vi "Error_And_Status_Test.vi"() -> ()   [LabVIEW 2017]
uses:
  Classes/ADCP.lvclass
panel:
  out "Test conditions / results":T1(array[cluster])
  in  "ADCP Session Parameters":T2
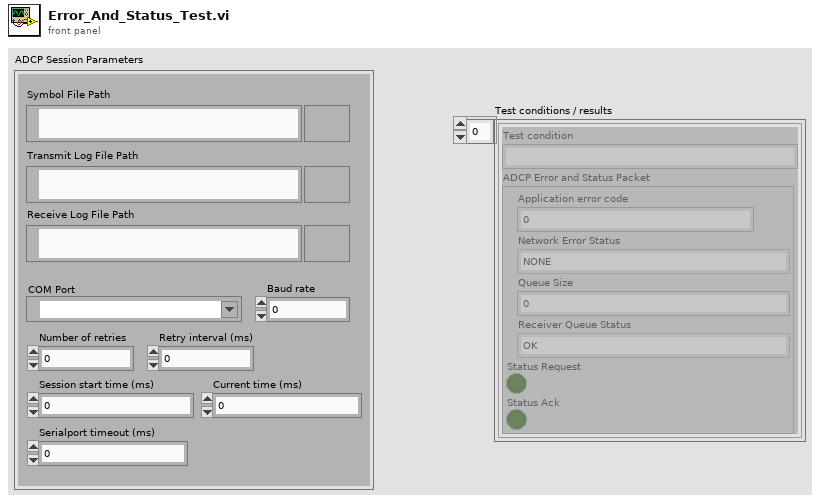
[diagram p1: front panel]
types:
  T1 = cluster{"Test condition":string, "ADCP Error and Status Packet":cluster{"Application error code":u16, "Network Error Status":enum16{"NONE", "CONNECTION_ALREADY_OPEN", "CONNECTION_ALREADY_CLOSED", "INVALID_FRAME_REQUEST"}, "Queue Size":u16, "Receiver Queue Status":enum16{"OK", "EMPTY", "FULL"}, "Status Request":bool, "Status Ack":bool}}[]
  T2 = cluster{"Symbol File Path":path, "Transmit Log File Path":path, "Receive Log File Path":path, "COM Port":refnum<visa-resource-name>, "Baud rate":u32, "Number of retries":u16, "Retry interval (ms)":u16, "Session start time (ms)":u32, "Current time (ms)":u32, "Serialport timeout (ms)":u32}
  T3 = cluster{"Application error code":u16, "Network Error Status":enum16{"NONE", "CONNECTION_ALREADY_OPEN", "CONNECTION_ALREADY_CLOSED", "INVALID_FRAME_REQUEST"}, "Queue Size":u16, "Receiver Queue Status":enum16{"OK", "EMPTY", "FULL"}, "Status Request":bool, "Status Ack":bool}
  T4 = cluster{"Application error code":u16, "Network Error Status":enum16{"NONE", "CONNECTION_ALREADY_OPEN", "CONNECTION_ALREADY_CLOSED", "INVALID_FRAME_REQUEST"}, "Queue Size":u16, "Receiver Queue Status":enum16{"OK", "EMPTY", "FULL"}, "Status Request":bool, "Status Ack":bool}[]
  T5 = cluster{"Test condition":string, "ADCP Error and Status Packet":cluster{"Application error code":u16, "Network Error Status":enum16{"NONE", "CONNECTION_ALREADY_OPEN", "CONNECTION_ALREADY_CLOSED", "INVALID_FRAME_REQUEST"}, "Queue Size":u16, "Receiver Queue Status":enum16{"OK", "EMPTY", "FULL"}, "Status Request":bool, "Status Ack":bool}}
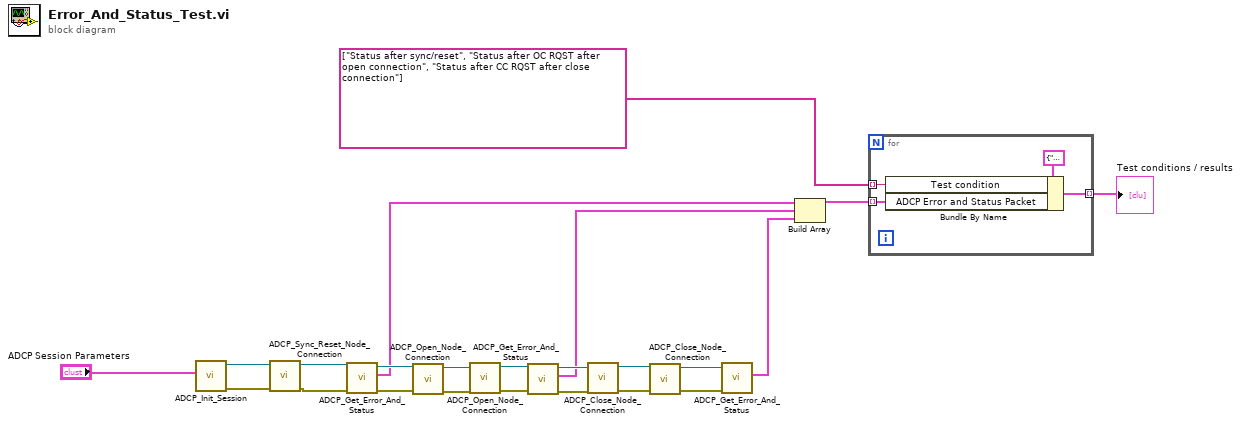
[diagram p0: block diagram]
diagram:
  n1 = call "ADCP_Init_Session.vi"("ADCP Session Parameters"="ADCP Session Parameters") -> ("error out"=w21:errorcluster, "ADCP out"=w22:refnum<class "ADCP.lvclass">)  [unwired: 9 in]
  n2 = call "ADCP_Sync_Reset_Node_Connection.vi"("error in (no error)"=w21, "ADCP In"=w22) -> ("error out"=w19:errorcluster, "ADCP Out"=w20:refnum<class "ADCP.lvclass">)  [unwired: 8 in]
  n3 = call "ADCP_Get_Error_And_Status.vi"("error in (no error)"=w19, "ADCP In"=w20) -> ("error out"=w17:errorcluster, "Error and Status"=w5:T3, "ADCP Out"=w18:refnum<class "ADCP.lvclass">)  [unwired: 7 in]
  n4 = call "ADCP_Open_Node_Connection.vi"("error in (no error)"=w17, "ADCP In"=w18) -> ("error out"=w15:errorcluster, "ADCP Out"=w16:refnum<class "ADCP.lvclass">)  [unwired: 8 in]
  n5 = call "ADCP_Open_Node_Connection.vi"("error in (no error)"=w15, "ADCP In"=w16) -> ("error out"=w13:errorcluster, "ADCP Out"=w14:refnum<class "ADCP.lvclass">)  [unwired: 8 in]
  n6 = call "ADCP_Get_Error_And_Status.vi"("error in (no error)"=w13, "ADCP In"=w14) -> ("error out"=w12:errorcluster, "Error and Status"=w4:T3, "ADCP Out"=w11:refnum<class "ADCP.lvclass">)  [unwired: 7 in]
  n7 = call "ADCP_Close_Node_Connection.vi"("error in (no error)"=w12, "ADCP In"=w11) -> ("error out"=w9:errorcluster, "ADCP Out"=w10:refnum<class "ADCP.lvclass">)  [unwired: 8 in]
  n8 = call "ADCP_Close_Node_Connection.vi"("error in (no error)"=w9, "ADCP In"=w10) -> ("error out"=w7:errorcluster, "ADCP Out"=w8:refnum<class "ADCP.lvclass">)  [unwired: 8 in]
  n9 = call "ADCP_Get_Error_And_Status.vi"("error in (no error)"=w7, "ADCP In"=w8) -> ("Error and Status"=w3:T3)  [unwired: 7 in, 2 out]
  n10 = Build Array(w5, w4, w3) -> (w2:T4)
  n11 = for {
    tunnel: [w26] -> w6 mode=indexing
    tunnel: w2 -> [w25] mode=indexing
    tunnel: string[] ["Status after sync/reset", "Status after OC RQST after open connection", "Status after CC RQST after close connection"] -> [w24] mode=indexing
    n12 = Bundle By Name(cluster=T5 {"Test condition"="", "ADCP Error and Status Packet"={"Application error code"=0, "Network Error Status"=enum."NONE", "Queue Size"=0, "Receiver Queue Status"=enum."OK", "Status Request"=FALSE, "Status Ack"=FALSE}}, "Test condition"=w24, "ADCP Error and Status Packet"=w25) -> (w26:T5)
  }
  "Test conditions / results" <- w6
